vi "Euler to Quaternion.vi"(0 "R1":dbl format="%#_13g", 1 "Rotation Order":T2=enum."ZXY, 312", 2 "R2":dbl format="%#_13g", 3 "R3":dbl format="%#_13g", 4 "Reference Frame":T1(ring)) -> (5 "quaternion":T3)   [LabVIEW 2016]
uses:
  <vilib>/robotics/Kinematics/Quaternion.ctl
  <userlib>/836-Libraries/Sensor/IMU/Rot Order.ctl
  <vilib>/Analysis/_algsub.llb/Vector Norm.vi
  <vilib>/Analysis/_algsub.llb/Real Vector Norm.vi
  <vilib>/robotics/Kinematics/NI_Kinematics.lvlib
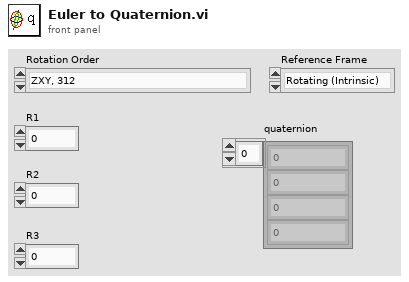
[diagram p1: front panel]
types:
  T1 = enum16{"Rotating (Intrinsic)", "Fixed (Extrinsic)"}
  T2 = typedef "Rot Order.ctl" = enum16{"ZXZ, 313", "XYX, 121", "YZY, 232", "ZYZ, 323", "XZX, 131", "YXY, 212", "XYZ, 123", "YZX, 231", "ZXY, 312", "XZY, 132", "ZYX, 321 NASA Standard Airplane", "YXZ, 213"}
  T3 = typedef "NI_Kinematics.lvlib/Quaternion.ctl" = dbl[]
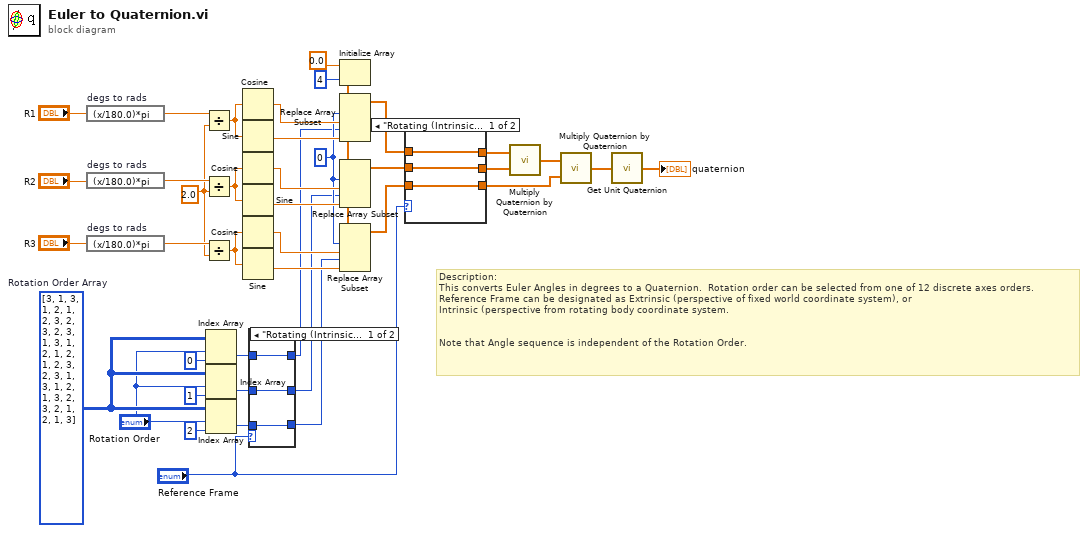
[diagram p0: block diagram]
diagram:
  w18 = i32[][] [[3, 1, 3], [1, 2, 1], [2, 3, 2], [3, 2, 3], [1, 3, 1], [2, 1, 2], [1, 2, 3], [2, 3, 1], [3, 1, 2], [1, 3, 2], [3, 2, 1], [2, 1, 3]]  # Rotation Order Array
  w37 = 2.0 ("y")
  w15 = 0 ("index")
  # "Description:\nThis converts Euler Angles in degrees to a Quaternion.  Rotation order can be selected from one of 12 discrete axes orders.\nReference Frame can be designated as Extrinsic (perspective of fixed world coordinate system), or\nIntrinsic (perspective from rotating body coordinate system.\n\n\nNote that Angle sequence is independent of the Rotation Order."
  n1 = expression code="(x/180.0)*pi" "degs to rads"("R1") -> (w39:dbl)
  n2 = expression code="(x/180.0)*pi" "degs to rads"("R2") -> (w40:dbl)
  n3 = expression code="(x/180.0)*pi" "degs to rads"("R3") -> (w41:dbl)
  n4 = Divide(x=w39, y=w37) -> (x/y=w27:dbl)
  n5 = Divide(x=w40, y=w37) -> (x/y=w32:dbl)
  n6 = Divide(x=w41, y=w37) -> (x/y=w33:dbl)
  n7 = Index Array(array=w18, index (row)="Rotation Order", index (col)=0 ("disabled index (col)")) -> (element=w9:i32)
  n8 = Index Array(array=w18, index (row)="Rotation Order", index (col)=1 ("disabled index (col)")) -> (element=w2:i32)
  n9 = Index Array(array=w18, index (row)="Rotation Order", index (col)=2 ("disabled index (col)")) -> (element=w8:i32)
  n10 = Cosine(x=w27) -> (cos(x)=w28:dbl)
  n11 = Sine(x=w27) -> (sin(x)=w29:dbl)
  n12 = Cosine(x=w32) -> (cos(x)=w31:dbl)
  n13 = Sine(x=w32) -> (sin(x)=w30:dbl)
  n14 = Cosine(x=w33) -> (cos(x)=w34:dbl)
  n15 = Sine(x=w33) -> (sin(x)=w35:dbl)
  n16 = case shown="\"Rotating (Intrinsic)\", Default" "Reference Frame" {
    tunnel: w9 -> [w44 w47]
    tunnel: w8 -> [w43 w46]
    tunnel: [w44 w46] -> w7
    tunnel: [w43 w47] -> w6
    tunnel: w2 -> [w42 w45]
    tunnel: [w42 w45] -> w1
    frame "Rotating (Intrinsic)", Default {
    }
    frame "Fixed (Extrinsic)" {
    }
  }
  n17 = Initialize Array(0.0 ("element"), 4 ("dimension size")) -> (w36:dbl[])
  n18 = Replace Array Subset(array=w36, new element #1=w28, index #1=w15, new element #2=w29, index #2=w7) -> (w24:dbl[])
  n19 = Replace Array Subset(array=w36, new element #1=w31, index #1=w15, new element #2=w30, index #2=w1) -> (w23:dbl[])
  n20 = Replace Array Subset(array=w36, new element #1=w34, index #1=w15, new element #2=w35, index #2=w6) -> (w22:dbl[])
  n21 = case shown="\"Rotating (Intrinsic)\", Default" "Reference Frame" {
    tunnel: [w50 w52] -> w12
    tunnel: w24 -> [w50 w51]
    tunnel: w23 -> [w49 w53]
    tunnel: w22 -> [w48 w52]
    tunnel: [w49 w53] -> w11
    tunnel: [w48 w51] -> w10
    frame "Rotating (Intrinsic)", Default {
    }
    frame "Fixed (Extrinsic)" {
    }
  }
  n22 = call <vilib>:"Multiply Quaternion by Quaternion.vi"("y"=w11, "quaternion"=w12) -> ("product"=w14:T3)
  n23 = call <vilib>:"Multiply Quaternion by Quaternion.vi"("y"=w10, "quaternion"=w14) -> ("product"=w13:T3)
  n24 = call <vilib>:"Get Unit Quaternion.vi"("quaternion"=w13) -> ("unit quaternion"=→"quaternion":T3)
